vi "Read FlowControlValveCompensator.vi"(11 "DualActingPneumaticCylinder in":refnum<class "DualActingPneumaticCylinder.lvclass">) -> (2 "FlowControlValveCompensator.lvclass":refnum<class "FlowControlValveCompensator.lvclass">, 3 "DualActingPneumaticCylinder out":refnum<class "DualActingPneumaticCylinder.lvclass">)   [LabVIEW 2013, in "DualActingPneumaticCylinder.lvclass"]
uses:
  DualActingPneumaticCylinder.lvclass
  FlowControlValveCompensator/FlowControlValveCompensator.lvclass
  DualActingPneumaticCylinder.lvclass/DualActingPneumaticCylinder.ctl
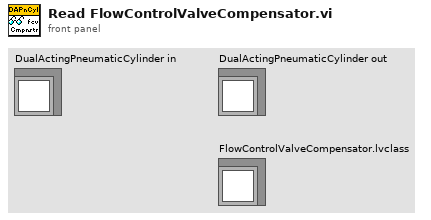
[diagram p1: front panel]
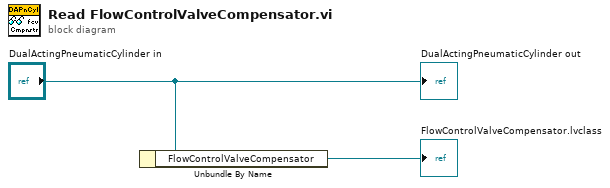
[diagram p0: block diagram]
diagram:
  n1 = Unbundle By Name("DualActingPneumaticCylinder in") -> ("FlowControlValveCompensator"=→"FlowControlValveCompensator.lvclass":refnum<class "FlowControlValveCompensator.lvclass">)
  "DualActingPneumaticCylinder out" <- "DualActingPneumaticCylinder in"
